vi "DSF.Engine.Transfer.Initialize.Channels Pointer.vi"(8 "error in (no error)":errorcluster, 10 "Device Ref in":T1=18446744073709551615 format="%.0x", 11 "Transfer in":refnum<class "DSF.Engine.Transfer.lvclass">) -> (0 "error out":errorcluster, 3 "Transfer out":refnum<class "DSF.Engine.Transfer.lvclass">)   [LabVIEW 2016, in "DSF.Engine.lvlib" / "DSF.Engine.Transfer.lvclass"]
uses:
  DSF.Engine.Transfer.lvclass
  <vilib>/NI Veristand/Custom Device API/Custom Device Item Ref.ctl
  DSF.Engine.Transfer.lvclass/DSF.Engine.Transfer.ctl
  Shared/Classes/Transfer/DSF.Shared.Configuration.Transfer.lvclass/DSF.Shared.Configuration.Transfer.ctl
  Shared/Classes/Transfer/DSF.Shared.Configuration.Transfer.Get Channel Descriptors.vi
  Shared/Classes/Transfer/DSF.Shared.Configuration.Transfer.Get Direction.vi
  Shared/Classes/Transfer/DSF.Shared.Configuration.Transfer.lvclass
  <vilib>/NI Veristand/Custom Device API/Custom Device API.lvlib
  Pointer/DSF.Engine.Pointer.VS Channels.lvclass
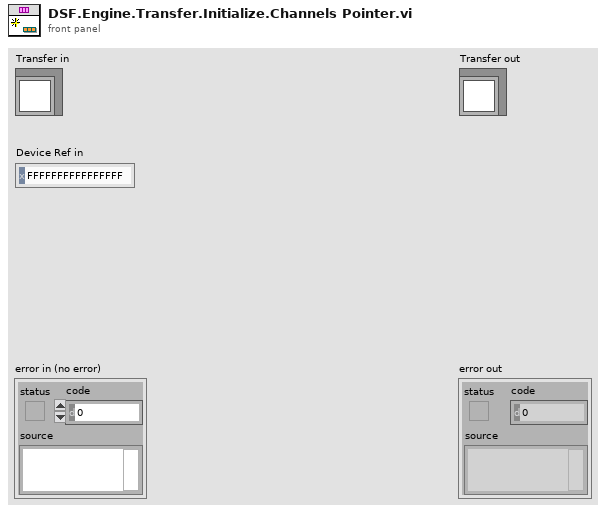
[diagram p1: front panel]
types:
  T1 = typedef "Custom Device API.lvlib/Custom Device Item Ref.ctl" = u64
  T2 = typedef "Custom Device API.lvlib/Data Access Type.ctl" = enum16{"Read", "Write"}
  T3 = typedef "DSF.Shared.lvlib/DSF.Shared.Typedefs.Configuration.Transfer.Channel Block Descriptor.ctl" = cluster{"First Channel Descriptor":T4, "count":u64, "vs channel index":u64}
  T4 = typedef "DSF.Shared.lvlib/DSF.Shared.Typedefs.Configuration.Transfer.Channel Descriptor.ctl" = cluster{"Channel Parameters":T5, "VS Channel Ref":T1}
  T5 = typedef "DSF.Shared.lvlib/DSF.Shared.Typedefs.Configuration.Transfer.Channel Parameters.ctl" = cluster{"offset":u64, "data type":T6}
  T6 = typedef "DSF.Shared.lvlib/DSF.Shared.Typedefs.Data Type.ctl" = enum8{"Bool", "SGL", "DBL", "I8", "I16", "I32", "I64", "U8", "U16", "U32", "U64"}
  T7 = typedef "Custom Device API.lvlib/Data Reference.ctl" = i32
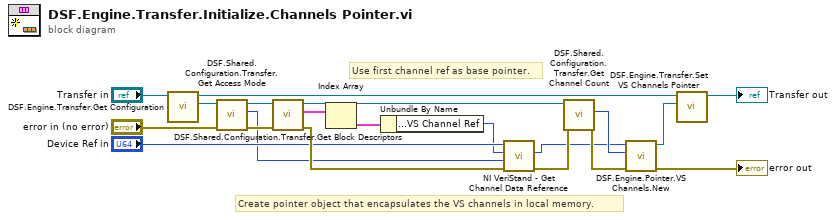
[diagram p0: block diagram]
diagram:
  # "Use first channel ref as base pointer."
  # "Create pointer object that encapsulates the VS channels in local memory."
  n1 = call "DSF.Engine.Transfer.Get Configuration.vi"("Transfer in"="Transfer in") -> ("Configuration"=w6:refnum<class "DSF.Shared.Configuration.Transfer.lvclass">, "Transfer out"=w5:refnum<class "DSF.Engine.Transfer.lvclass">)  [unwired: 9 in]
  n2 = call "DSF.Shared.Configuration.Transfer.Get Access Mode.vi"("error in (no error)"="error in (no error)", "Transfer Configuration in"=w6) -> ("error out"=w8:errorcluster, "Access"=w7:T2, "Transfer Configuration out"=w9:refnum<class "DSF.Shared.Configuration.Transfer.lvclass">)  [unwired: 7 in]
  n3 = call "DSF.Shared.Configuration.Transfer.Get Block Descriptors.vi"("error in (no error)"=w8, "Transfer Configuration in"=w9) -> ("error out"=w19:errorcluster, "Channel Blocks"=w17:T3[], "Transfer Configuration out"=w14:refnum<class "DSF.Shared.Configuration.Transfer.lvclass">)  [unwired: 7 in]
  n4 = Index Array(array=w17) -> (element=w16:T3)  [unwired: 1 in]
  n5 = Unbundle By Name(w16) -> ("First Channel Descriptor.VS Channel Ref"=w15:T1)
  n6 = call <vilib>:"NI VeriStand - Get Channel Data Reference.vi"("error in (no error)"=w19, "Access"=w7, "Channel Ref in"=w15, "Device Ref in"="Device Ref in") -> ("error out"=w12:errorcluster, "Channel Data Reference"=w10:T7)  [unwired: 5 in, 1 out]
  n7 = call "DSF.Shared.Configuration.Transfer.Get Channel Count.vi"("error in (no error)"=w12, "Transfer Configuration in"=w14) -> ("error out"=w11:errorcluster, "channel count"=w13:u64)  [unwired: 7 in, 1 out]
  n8 = call "DSF.Engine.Pointer.VS Channels.New.vi"("error in (no error)"=w11, "channel count"=w13, "Data Reference"=w10) -> ("error out"=→"error out":errorcluster, "VS Channels Pointer out"=w1:refnum<class "DSF.Engine.Pointer.VS Channels.lvclass">)  [unwired: 7 in]
  n9 = call "DSF.Engine.Transfer.Set VS Channels Pointer.vi"("VS Channels Pointer"=w1, "Transfer in"=w5) -> ("Transfer out"=→"Transfer out":refnum<class "DSF.Engine.Transfer.lvclass">)  [unwired: 9 in]
